vi "Clean (After).vi"() -> ()   [LabVIEW 2010]
doc: "A sample VI demonstrating a cleaned up front panel and block diagram."
panel:
  in  "Math Functions":enum32{"Add", "Multiply"}(tab)
  in  "Value X":dbl
  in  "Value Y":dbl
  out "Result":dbl
  in  "Value X":dbl
  in  "Value Y":dbl
  out "Result":dbl
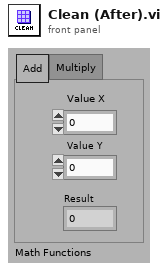
[diagram p1: front panel]
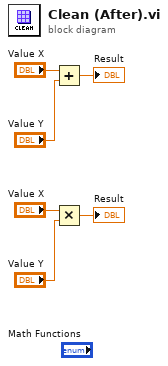
[diagram p0: block diagram]
diagram:
  n1 = Add(x="Value X", y="Value Y") -> (x+y=→"Result":dbl)
  n2 = Multiply(x="Value X", y="Value Y") -> (x*y=→"Result":dbl)
